vi "Error Strings.vi"() -> ()   [LabVIEW 2016, in "Scan Engine Custom Device.lvlib"]
uses:
  Scan Engine Custom Device.lvlib
panel:
  out "537717":string
  out "537716":string
  out "537715":string
  out "537714":string="Timeout communicating with EtherCAT reconfiguration loop."
  out "537713":string="ECAT Slave I/O Varaible \"%s\" does not match configuration to SDF \"%s\"."
  out "537712":string
  out "537711":string
  out "537710":string
  out "537709":string
  out "537708":string
  out "537707":string="UDV container not found."
  out "537706":string="The EtherCAT slave \"%s\" configuration does not match the currently deployed FPGA personality."
  out "537705":string="UDV \"%s\" not found."
  out "537704":string="Timeout communicating with asyncronyous loop."
  out "537703":string="Asynchronous loop in unexpected state."
  out "537702":string="Module \"%s\" (slot %d) not found."
  out "537701":string="EtherCAT slave %d not found."
  out "537700":string="EtherCAT master %d not found."
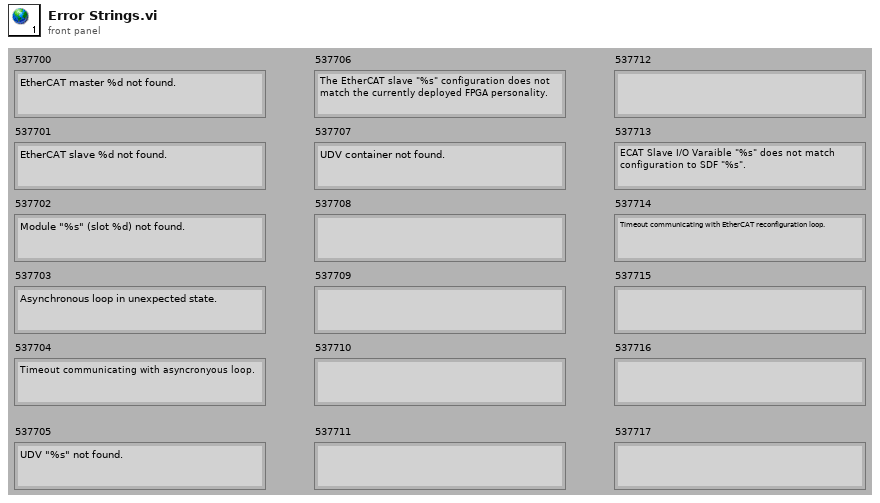
[diagram p1: front panel]
diagram:
